vi "Momentary_Switch.vi"(10 "Rise/Fall (Rise = T)":bool, 11 "in":bool) -> (3 "out":bool)   [LabVIEW 2014]
panel:
  # "This subystem turns a button push into a momentary switch"
  # "Rise/fall  = True (will detect rise)\n                    False (detects fall)"
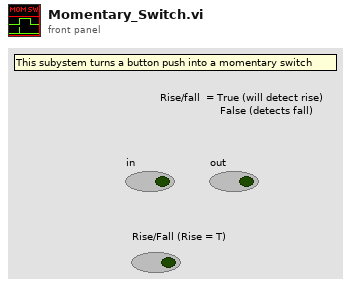
[diagram p1: front panel]
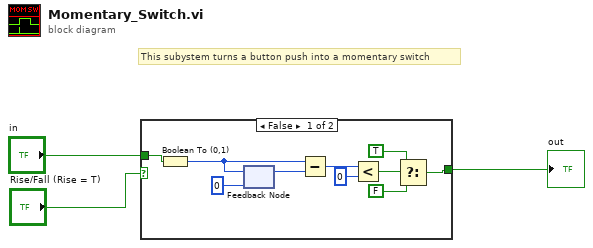
[diagram p0: block diagram]
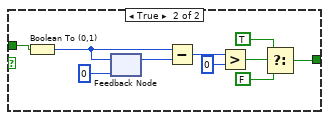
[diagram p2: hidden frame]
diagram:
  # "This subystem turns a button push into a momentary switch"
  n1 = case shown="False" "Rise/Fall (Rise = T)" {
    tunnel: [w5 w23] -> w3
    tunnel: "in" -> [w4 w17]
    frame False {
      n2 = Boolean To (0,1)(Boolean=w4) -> (0, 1=w8:i16)
      n3 = feedback #1(0) -> (w9:i32)
      n4 = feedback-in #1(w8) -> ()
      n5 = Subtract(x=w8, y=w9) -> (x-y=w10:i32)
      n6 = Less?(x=w10, y=0) -> (x < y?=w11:bool)
      n7 = Select(t=TRUE, s=w11, f=FALSE) -> (s? t:f=w5:bool)
    }
    frame True {
      n8 = Boolean To (0,1)(Boolean=w17) -> (0, 1=w16:i16)
      n9 = feedback #2(0) -> (w18:i32)
      n10 = feedback-in #2(w16) -> ()
      n11 = Subtract(x=w16, y=w18) -> (x-y=w19:i32)
      n12 = Greater?(x=w19, y=0) -> (0:w20:bool)
      n13 = Select(t=TRUE, s=w20, f=FALSE) -> (s? t:f=w23:bool)
    }
  }
  "out" <- w3
